vi "Generate license file for this machine.vi"(8 "error in (no error)":errorcluster, 10 "prefix text":string="tctechinc", 11 "folder path":path) -> (0 "error out":errorcluster, 3 "file path":path)   [LabVIEW 2016]
doc: "Generate license file with the information of local MAC address and the <b>prefix text</b>. The <b>folder path</b> is assigned as the container of the license file in the <b>file path</b>. If the <b>folder path</b> is empty, the license file is generated and located in the same folder as this VI."
panel:
  out "MD5 Message Digest":string
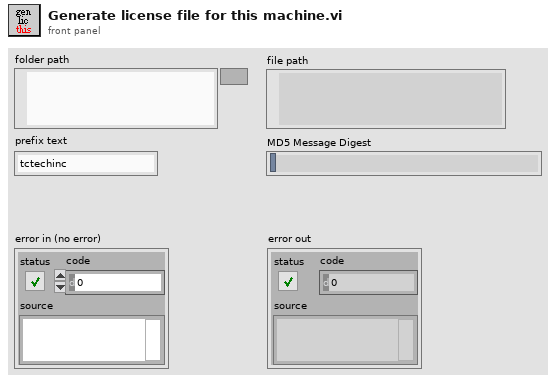
[diagram p1: front panel]
types:
  T1 = enum16{"open", "replace", "create", "open or create", "replace or create", "replace or create with confirmation"}
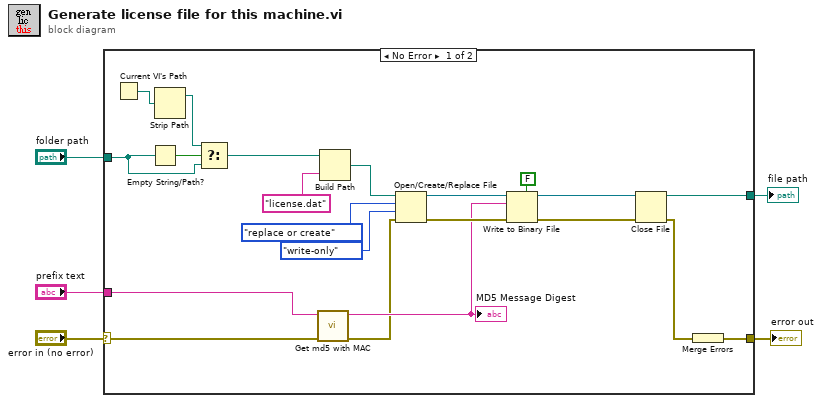
[diagram p0: block diagram]
diagram:
  n1 = case shown="No Error" "error in (no error)" {
    selector: "error in (no error)" -> [w16 w27]
    tunnel: [w18 _] -> w5
    tunnel: [w14 w27] -> w3
    tunnel: "prefix text" -> [w17 _]
    tunnel: "folder path" -> [w8 _]
    frame No Error {
      n2 = Current VI's Path() -> (path=w11:path)
      n3 = Empty String/Path?(string/path=w8) -> (empty?=w10:bool)
      n4 = Strip Path(path=w11) -> (stripped path=w9:path)  [unwired: 1 out]
      n5 = Select(t=w9, s=w10, f=w8) -> (s? t:f=w7:path)
      n6 = call "Get md5 with MAC.vi"("error in (no error)"=w16, "prefix text"=w17) -> ("error out"=w6:errorcluster, "MD5 Message Digest"=w13:string)  [unwired: 8 in]
      "MD5 Message Digest" <- w13
      n7 = Build Path(base path=w7, name or relative path="license.dat") -> (appended path=w21:path)
      n8 = Open/Create/Replace File(file path (use dialog)=w21, error in=w6, operation (0:open)=T1."replace or create", access (0:read/write)=enum16{"read/write", "read-only", "write-only"}."write-only") -> (refnum out=w25:refnum<file>, error out=w24:errorcluster)  [unwired: 2 in, 1 out]
      n9 = Write to Binary File(file (use dialog)=w25, data=w13, error in=w24, 5:FALSE ("prepend array or string size? (T)")) -> (refnum out=w23:refnum<file>, error out=w22:errorcluster)  [unwired: 2 in, 1 out]
      n10 = Close File(refnum=w23, error in=w22) -> (path=w18:path, error out=w15:errorcluster)
      n11 = Merge Errors(w15) -> (w14:errorcluster)
    }
    frame Error {
    }
  }
  "error out" <- w3
  "file path" <- w5
